vi "ARRAY3DHandle.vi"() -> ()   [LabVIEW 2014]
doc: "This function sums each element in pages 0 through n-2 of an n page sized 3-D array and places the values in the corresponding element on page n-1. It is assumed that page n-1 is already allocated in the input array.\n\nFor information on the data types used for the DLL function, right-click on the Call Library Function node and choose Configure."
uses:
  CLF_Example.dll
panel:
  out "output":dbl[][][](array[numeric])
  in  "input":dbl[][][](array[numeric])=[[[0.0, 1.0], [2.0, 3.0], [4.0, 5.0], [6.0, 7.0]], [[0.0, 2.0], [4.0, 6.0], [8.0, 10.0], [12.0, 14.0]], [[0.0, 0.0], [0.0, 0.0], [0.0, 0.0], [0.0, 0.0]], [[0.0, 1.0], [2.0, 3.0], [4.0, 5.0], [6.0, 7.0]]]
  # "See the block diagram for more information."
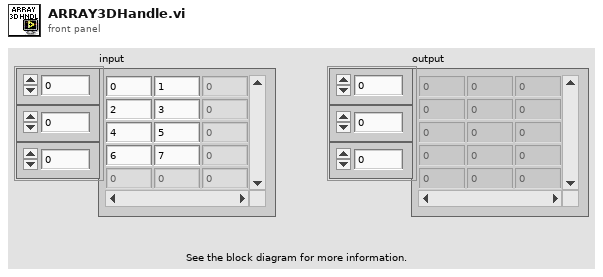
[diagram p1: front panel]
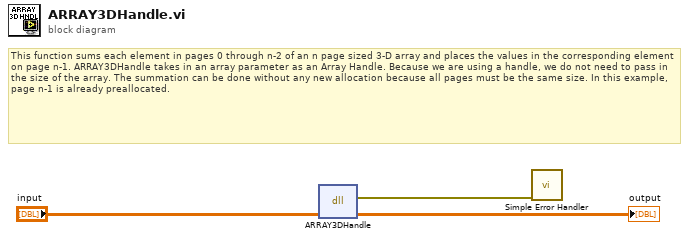
[diagram p0: block diagram]
diagram:
  # "This function sums each element in pages 0 through n-2 of an n page sized 3-D array and places the values in the corresponding element on page n-1. ARRAY3DHandle takes in an array parameter as an Array Handle. Because we are using a handle, we do not need to pass in the size of the array. The summation can be done without any new allocation because all pages must be the same size. In this example, page n-1 is already preallocated."
  n1 = dll-call lib="e:/builds/penguin/labview/branches/2014/dev/dist/examples/Connectivity/Libraries and Executables/DLL Calling VIs/CLF_Example**.*" fn="ARRAY3DHandle"("array"="input") -> (error out=w1:errorcluster, "array"=→"output":dbl[][][])  [unwired: 3 in, 2 out]
  n2 = call <vilib>:"Simple Error Handler.vi"("error in (no error)"=w1) -> ()  [unwired: 4 in, 5 out]
